vi "forma número complejo.vi"(9 "k":dbl, 11 "n":dbl) -> (3 "n + ik":cdb)   [LabVIEW 2013]
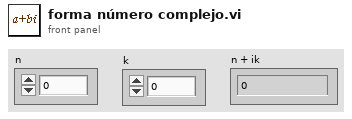
[diagram p1: front panel]
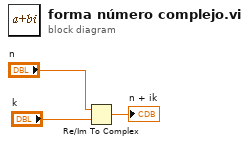
[diagram p0: block diagram]
diagram:
  n1 = Re/Im To Complex(1:"k", 2:"n") -> (0:→"n + ik":cdb)
